vi "OpenALPR_Recognise.vi"(8 "error in (no error)":errorcluster, 11 "img":string) -> (0 "error out":errorcluster, 2 "Detected plates":string, 3 "img out":string)   [LabVIEW 2014, in "OpenALPR in LabView.lvlib"]
doc: "Rcognise all plates in a image.\n\n!!! YOU HAVE TO HAVE A \"OPENALPR_PATH\" ENVIRONMENT VARIABLE WITH THE \"openalpr_32\" DIRECTORY WITCH CONTAINS THE CONFIG FILE AND THE RUNTIME DIRECTORY TO THE SUCCELFUL LOAD! !!!\n\n\n\n\n\n\nextern \"C\" __declspec(dllexport) char* OALPRLabVIEW_Recognise(char* img);"
uses:
  OpenALPR in LabView.lvlib
  Dlls/OALPRLabVIEW.dll
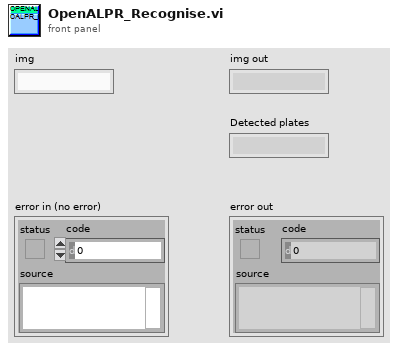
[diagram p1: front panel]
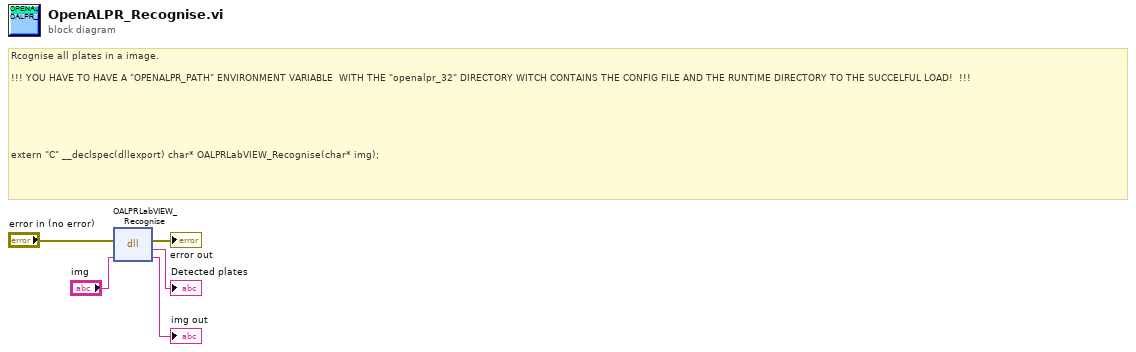
[diagram p0: block diagram]
diagram:
  # "Rcognise all plates in a image.\n\n!!! YOU HAVE TO HAVE A \"OPENALPR_PATH\" ENVIRONMENT VARIABLE  WITH THE \"openalpr_32\" DIRECTORY WITCH CONTAINS THE CONFIG FILE AND THE RUNTIME DIRECTORY TO THE SUCCELFUL LOAD!  !!!\n\n\n\n\n\n\nextern \"C\" __declspec(dllexport) char* OALPRLabVIEW_Recognise(char* img);"
  n1 = dll-call lib="PTH2abs EFelhasznÃ¡lÃ³kPixelbetyÃ¡rDesktopC19 -C3 Verseny bekÃ¼ldÃ©shez\tSmartMarkOpenALPR to LVOpenALPR_LabVIEWDllsOALPRLabVIEW.*" fn="OALPRLabVIEW_Recognise"(error in="error in (no error)", "img"="img") -> (error out=→"error out":errorcluster, "return type"=→"Detected plates":string, "img"=→"img out":string)  [unwired: 2 in, 1 out]
